vi "Read track.vi"() -> ()   [LabVIEW 2017]
panel:
  out "value":T1(array[cluster])
  out "text":string="[\n  {\n    \"Warning\": false,\n    \"Caption\": \"Dublin\",\n    \"Latitude_deg\": 6.3,\n    \"Longitude_deg\": 53.3,\n    \"Altitude_m\": 166.0,\n    \"Speed_m_s\": 66.0,\n    \"Temperature_C\": 28.3\n  },\n  {\n    \"Warning\": false,\n    \"Caption\": \"Galway\",\n    \"Latitude_deg\": 9.1,\n    \"Longitude_deg\": 53.3,\n    \"Altitude_m\": 270.0,\n    \"Speed_m_s\": 62.0,\n    \"Temperature_C\": 26.0\n  },\n  {\n    \"Warning\": false,\n    \"Caption\": \"Belfast\",\n    \"Latitude_deg\": 5.9,\n    \"Longitude_deg\": 54.6,\n    \"Altitude_m\": 224.0,\n    \"Speed_m_s\": 62.0,\n    \"Temperature_C\": 25.7\n  },\n  {\n    \"Warning\": false,\n    \"Caption\": \"Birmingham\",\n    \"Latitude_deg\": 1.9,\n    \"Longitude_deg\": 52.4,\n    \"Altitude_m\": 141.0,\n    \"Speed_m_s\": 65.0,\n    \"Temperature_C\": 32.1\n  },\n  {\n    \"Warning\": false,\n    \"Caption\": \"Bristol\",\n    \"Latitude_deg\": 2.6,\n    \"Longitude_deg\": 51.5,\n    \"Altitude_m\": 142.0,\n    \"Speed_m_s\": 69.0,\n    \"Temperature_C\": 33.2\n  },\n  {\n    \"Warning\": false,\n    \"Caption\": \"Leeds\",\n    \"Latitude_deg\": 1.5,\n    \"Longitude_deg\": 53.8,\n    \"Altitude_m\": 166.0,\n    \"Speed_m_s\": 60.0,\n    \"Temperature_C\": 30.2\n  },\n  {\n    \"Warning\": false,\n    \"Caption\": \"Liverpool\",\n    \"Latitude_deg\": 3.0,\n    \"Longitude_deg\": 53.4,\n    \"Altitude_m\": 229.0,\n    \"Speed_m_s\": 68.0,\n    \"Temperature_C\": 33.7\n  },\n  {\n    \"Warning\": false,\n    \"Caption\": \"London\",\n    \"Latitude_deg\": 0.1,\n    \"Longitude_deg\": 51.5,\n    \"Altitude_m\": 201.0,\n    \"Speed_m_s\": 64.0,\n    \"Temperature_C\": 33.7\n  },\n  {\n    \"Warning\": false,\n    \"Caption\": \"Manchester\",\n    \"Latitude_deg\": 2.3,\n    \"Longitude_deg\": 53.5,\n    \"Altitude_m\": 119.0,\n    \"Speed_m_s\": 67.0,\n    \"Temperature_C\": 26.3\n  },\n  {\n    \"Warning\": false,\n    \"Caption\": \"Newcastle-on-Tyne\",\n    \"Latitude_deg\": 1.6,\n    \"Longitude_deg\": 55.0,\n    \"Altitude_m\": 173.0,\n    \"Speed_m_s\": 66.0,\n    \"Temperature_C\": 26.0\n  },\n  {\n    \"Warning\": false,\n    \"Caption\": \"Plymouth\",\n    \"Latitude_deg\": 4.1,\n    \"Longitude_deg\": 50.4,\n    \"Altitude_m\": 167.0,\n    \"Speed_m_s\": 68.0,\n    \"Temperature_C\": 29.6\n  },\n  {\n    \"Warning\": false,\n    \"Caption\": \"Aberdeen\",\n    \"Latitude_deg\": 2.2,\n    \"Longitude_deg\": 57.2,\n    \"Altitude_m\": 213.0,\n    \"Speed_m_s\": 64.0,\n    \"Temperature_C\": 30.1\n  },\n  {\n    \"Warning\": false,\n    \"Caption\": \"Edinburgh\",\n    \"Latitude_deg\": 3.2,\n    \"Longitude_deg\": 55.9,\n    \"Altitude_m\": 132.0,\n    \"Speed_m_s\": 64.0,\n    \"Temperature_C\": 27.0\n  },\n  {\n    \"Warning\": false,\n    \"Caption\": \"Glasgow\",\n    \"Latitude_deg\": 4.3,\n    \"Longitude_deg\": 55.8,\n    \"Altitude_m\": 173.0,\n    \"Speed_m_s\": 60.0,\n    \"Temperature_C\": 28.8\n  },\n  {\n    \"Warning\": false,\n    \"Caption\": \"Amsterdam\",\n    \"Latitude_deg\": 4.9,\n    \"Longitude_deg\": 52.4,\n    \"Altitude_m\": 129.0,\n    \"Speed_m_s\": 69.0,\n    \"Temperature_C\": 29.3\n  },\n  {\n    \"Warning\": false,\n    \"Caption\": \"Rotterdam\",\n    \"Latitude_deg\": 4.5,\n    \"Longitude_deg\": 51.9,\n    \"Altitude_m\": 286.0,\n    \"Speed_m_s\": 68.0,\n    \"Temperature_C\": 27.6\n  },\n  {\n    \"Warning\": false,\n    \"Caption\": \"Den Haag\",\n    \"Latitude_deg\": 4.3,\n    \"Longitude_deg\": 52.1,\n    \"Altitude_m\": 187.0,\n    \"Speed_m_s\": 63.0,\n    \"Temperature_C\": 34.8\n  },\n  {\n    \"Warning\": false,\n    \"Caption\": \"Groningen\",\n    \"Latitude_deg\": 6.6,\n    \"Longitude_deg\": 53.2,\n    \"Altitude_m\": 120.0,\n    \"Speed_m_s\": 60.0,\n    \"Temperature_C\": 29.9\n  },\n  {\n    \"Warning\": false,\n    \"Caption\": \"Antwerpe\",\n    \"Latitude_deg\": 4.4,\n    \"Longitude_deg\": 51.2,\n    \"Altitude_m\": 197.0,\n    \"Speed_m_s\": 68.0,\n    \"Temperature_C\": 26.9\n  },\n  {\n    \"Warning\": false,\n    \"Caption\": \"Brussels\",\n    \"Latitude_deg\": 4.4,\n    \"Longitude_deg\": 50.9,\n    \"Altitude_m\": 193.0,\n    \"Speed_m_s\": 67.0,\n    \"Temperature_C\": 30.4\n  },\n  {\n    \"Warning\": false,\n    \"Caption\": \"Gent\",\n    \"Latitude_deg\": 3.7,\n    \"Longitude_deg\": 51.1,\n    \"Altitude_m\": 294.0,\n    \"Speed_m_s\": 62.0,\n    \"Temperature_C\": 31.8\n  },\n  {\n    \"Warning\": false,\n    \"Caption\": \"Oostende\",\n    \"Latitude_deg\": 2.9,\n    \"Longitude_deg\": 51.2,\n    \"Altitude_m\": 294.0,\n    \"Speed_m_s\": 68.0,\n    \"Temperature_C\": 31.6\n  },\n  {\n    \"Warning\": false,\n    \"Caption\": \"Brest\",\n    \"Latitude_deg\": 4.5,\n    \"Longitude_deg\": 48.4,\n    \"Altitude_m\": 151.0,\n    \"Speed_m_s\": 66.0,\n    \"Temperature_C\": 30.3\n  },\n  {\n    \"Warning\": false,\n    \"Caption\": \"Calais\",\n    \"Latitude_deg\": 1.9,\n    \"Longitude_deg\": 51.0,\n    \"Altitude_m\": 162.0,\n    \"Speed_m_s\": 61.0,\n    \"Temperature_C\": 31.3\n  },\n  {\n    \"Warning\": false,\n    \"Caption\": \"Paris\",\n    \"Latitude_deg\": 2.3,\n    \"Longitude_deg\": 48.8,\n    \"Altitude_m\": 163.0,\n    \"Speed_m_s\": 62.0,\n    \"Temperature_C\": 33.0\n  },\n  {\n    \"Warning\": false,\n    \"Caption\": \"Copenhagen\",\n    \"Latitude_deg\": 12.6,\n    \"Longitude_deg\": 55.7,\n    \"Altitude_m\": 197.0,\n    \"Speed_m_s\": 63.0,\n    \"Temperature_C\": 30.1\n  },\n  {\n    \"Warning\": false,\n    \"Caption\": \"Minsk\",\n    \"Latitude_deg\": 53.8,\n    \"Longitude_deg\": 27.6,\n    \"Altitude_m\": 186.0,\n    \"Speed_m_s\": 61.0,\n    \"Temperature_C\": 33.9\n  }\n]"
  in  "file (use dialog)":path=path "../tracks/track.json"
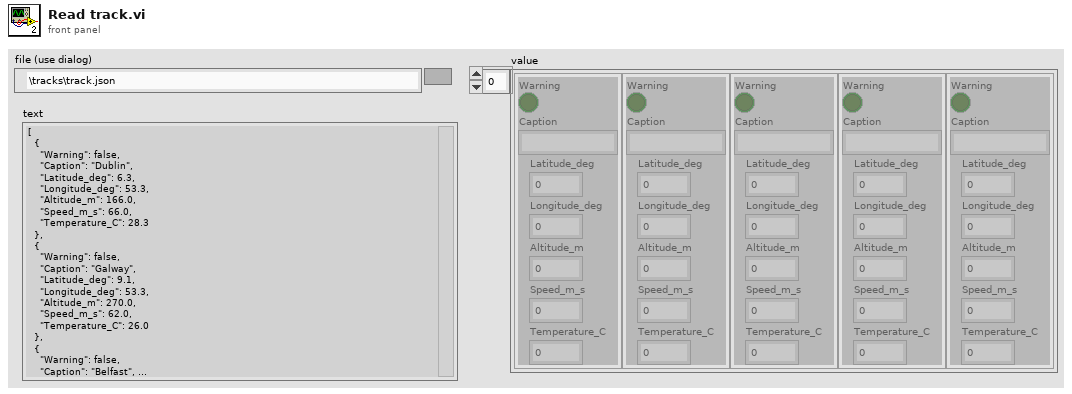
[diagram p1: front panel]
types:
  T1 = cluster{"Warning":bool, "Caption":string, "Latitude_deg":dbl, "Longitude_deg":dbl, "Altitude_m":dbl, "Speed_m_s":dbl, "Temperature_C":dbl}[]
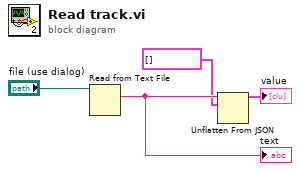
[diagram p0: block diagram]
diagram:
  n1 = Read from Text File(file (use dialog)="file (use dialog)") -> (text=w3:string)  [unwired: 3 in, 3 out]
  "text" <- w3
  n2 = Unflatten From JSON(JSON string=w3, type and defaults=T1 []) -> (value=→"value":T1)  [unwired: 5 in, 1 out]
